vi "Launch Tester.vi"   [LabVIEW 2020, in "Business Logic Tester.lvlib"]
uses:
  Business Logic Tester.lvlib
  Business Logic Tester/Business Logic Tester.lvclass
  C:/Program Files (x86)/National Instruments/LabVIEW 2020/vi.lib/ActorFramework/Actor/Actor.lvclass
  <vilib>/ActorFramework/Actor/Actor.lvclass
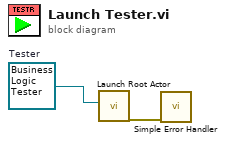
[diagram p0: block diagram]
diagram:
  w2 = refnum<class "Business Logic Tester.lvclass"> refnum  # Tester
  n1 = call <vilib>:"Launch Root Actor.vi"("Actor"=w2) -> ("error out"=w1:errorcluster)  [unwired: 9 in, 1 out]
  n2 = call <vilib>:"Simple Error Handler.vi"("error in (no error)"=w1) -> ()  [unwired: 4 in, 5 out]
